vi "DatastructureTest.vi"() -> ()   [LabVIEW 2013, in "VI-Test.lvlib"]
uses:
  lib/VI-Test.lvlib
  classes/Datastructure/Report/Report.lvclass
  classes/Datastructure/Norm/Norm.lvclass
  classes/Datastructure/Test/Test.lvclass
  classes/Datastructure/Image/img.lvclass
  classes/Datastructure/Setup/Setup.lvclass
  classes/Datastructure/Device/Device.lvclass
  Main/controls/Data.ctl
  Main/controls/State.ctl
  classes/Devices/emTestCWS500N/EMTestCWS500N.lvclass
  classes/Devices/CEG4500/CEG4500.lvclass
  classes/Devices/Tektronix RSA5106A/Tektronix RSA5106A.lvclass
  classes/Devices/DeviceInterface/Devices.ctl
  classes/Tests/TestInterface/Tests.ctl
  lib/XML.lvlib
  lib/TreeRepresentation.lvlib
panel:
  in  "gelesen von XML":string(tree)
  in  "gelesen vom Baum":string(tree)
  out "Fehler (Ausgang)":errorcluster
  in  "gelesen von Datenstruktur":string(tree)
  out "Report (Ausgang)":refnum<class "Report.lvclass">
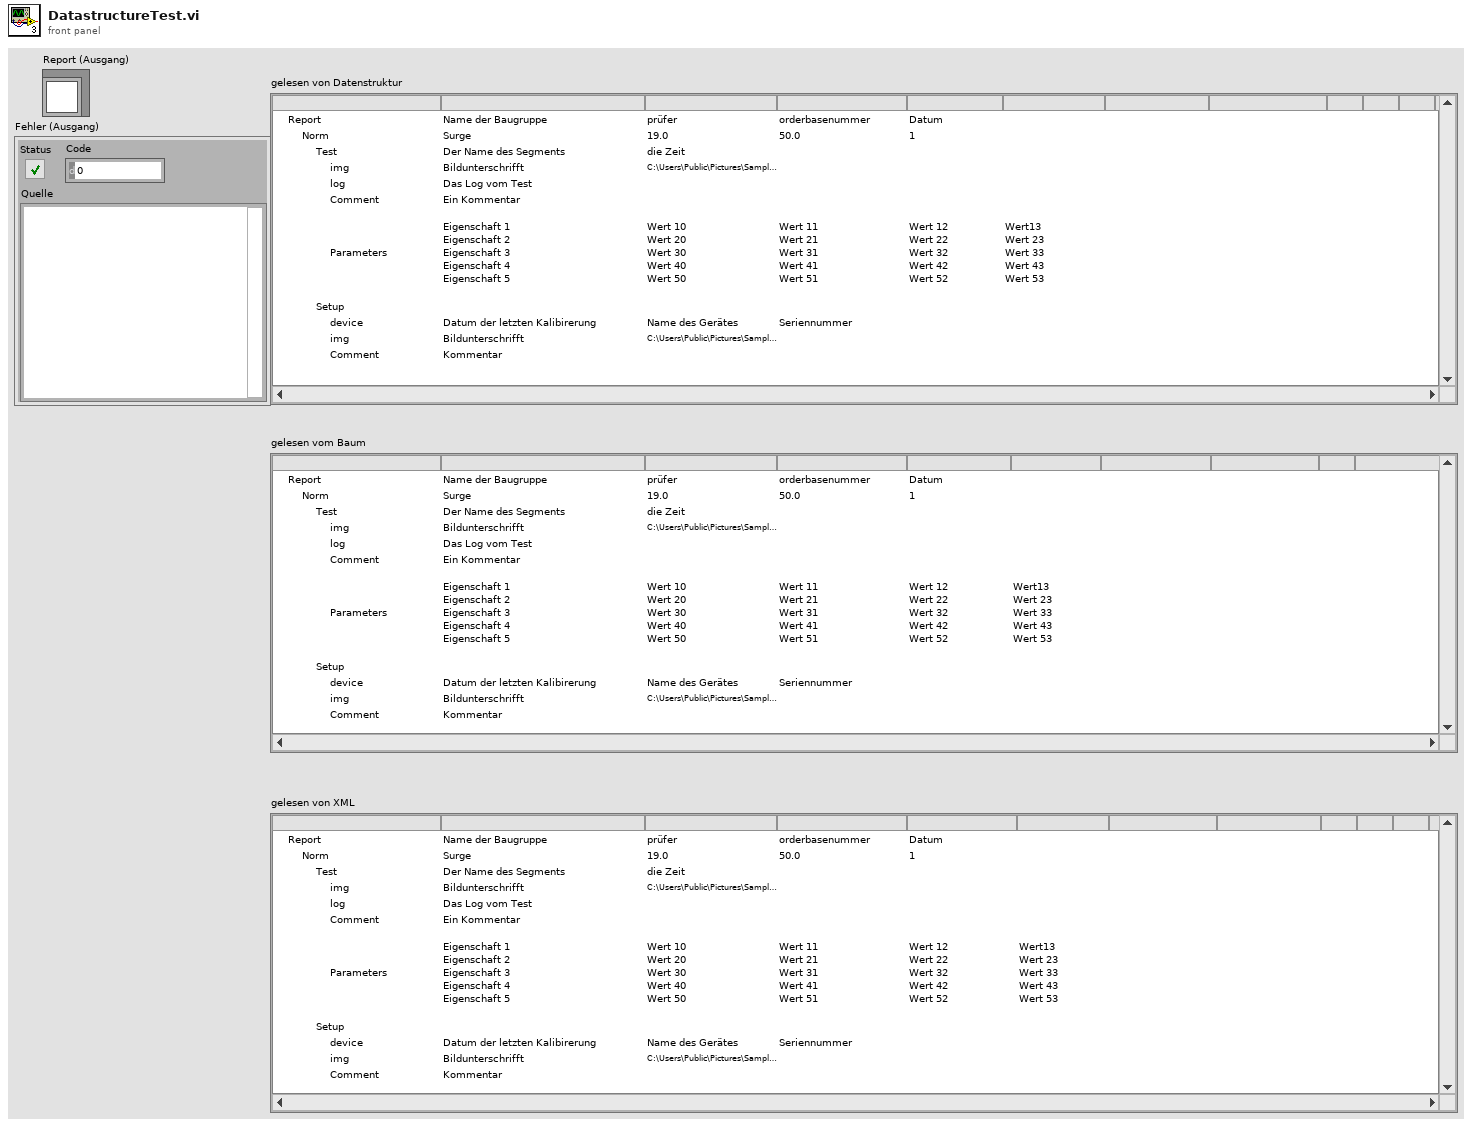
[diagram p1: front panel]
types:
  T1 = typedef "Data.ctl" = cluster{"Report.lvclass":refnum<class "Report.lvclass">, "Norm":string, "last State":T2, "Norm ID":i32, "parameter":string[][], "EMTestCWS500N.lvclass":refnum<class "EMTestCWS500N.lvclass">, "CEG4500.lvclass":refnum<class "CEG4500.lvclass">, "Tektronix RSA5106A.lvclass":refnum<class "Tektronix RSA5106A.lvclass">, "erfolgreich":bool, "log":string, "Kommentar":string, "Device Enum":T3, "Test Enum":T4, "debug":bool}
  T2 = typedef "State.ctl" = enum16{"create Pdf", "load Report", "save Report", "do Test", "CDN Kalibrierung", "enter Report Parameters", "new Test", "Protokoll", "read Tree", "update Tree", "Fehler", "Initialize", "Wait for Event", "Exit"}
  T3 = typedef "Devices.ctl" = enum16{"unbekannt", "Tektronix RSA5106A", "emTestCWS500N", "CEG-4500"}
  T4 = typedef "Tests.ctl" = enum16{"unbekannt", "Störaussendung", "Burst", "ESD", "Surge", "Spannungseinbruch", "HF-Felder"}
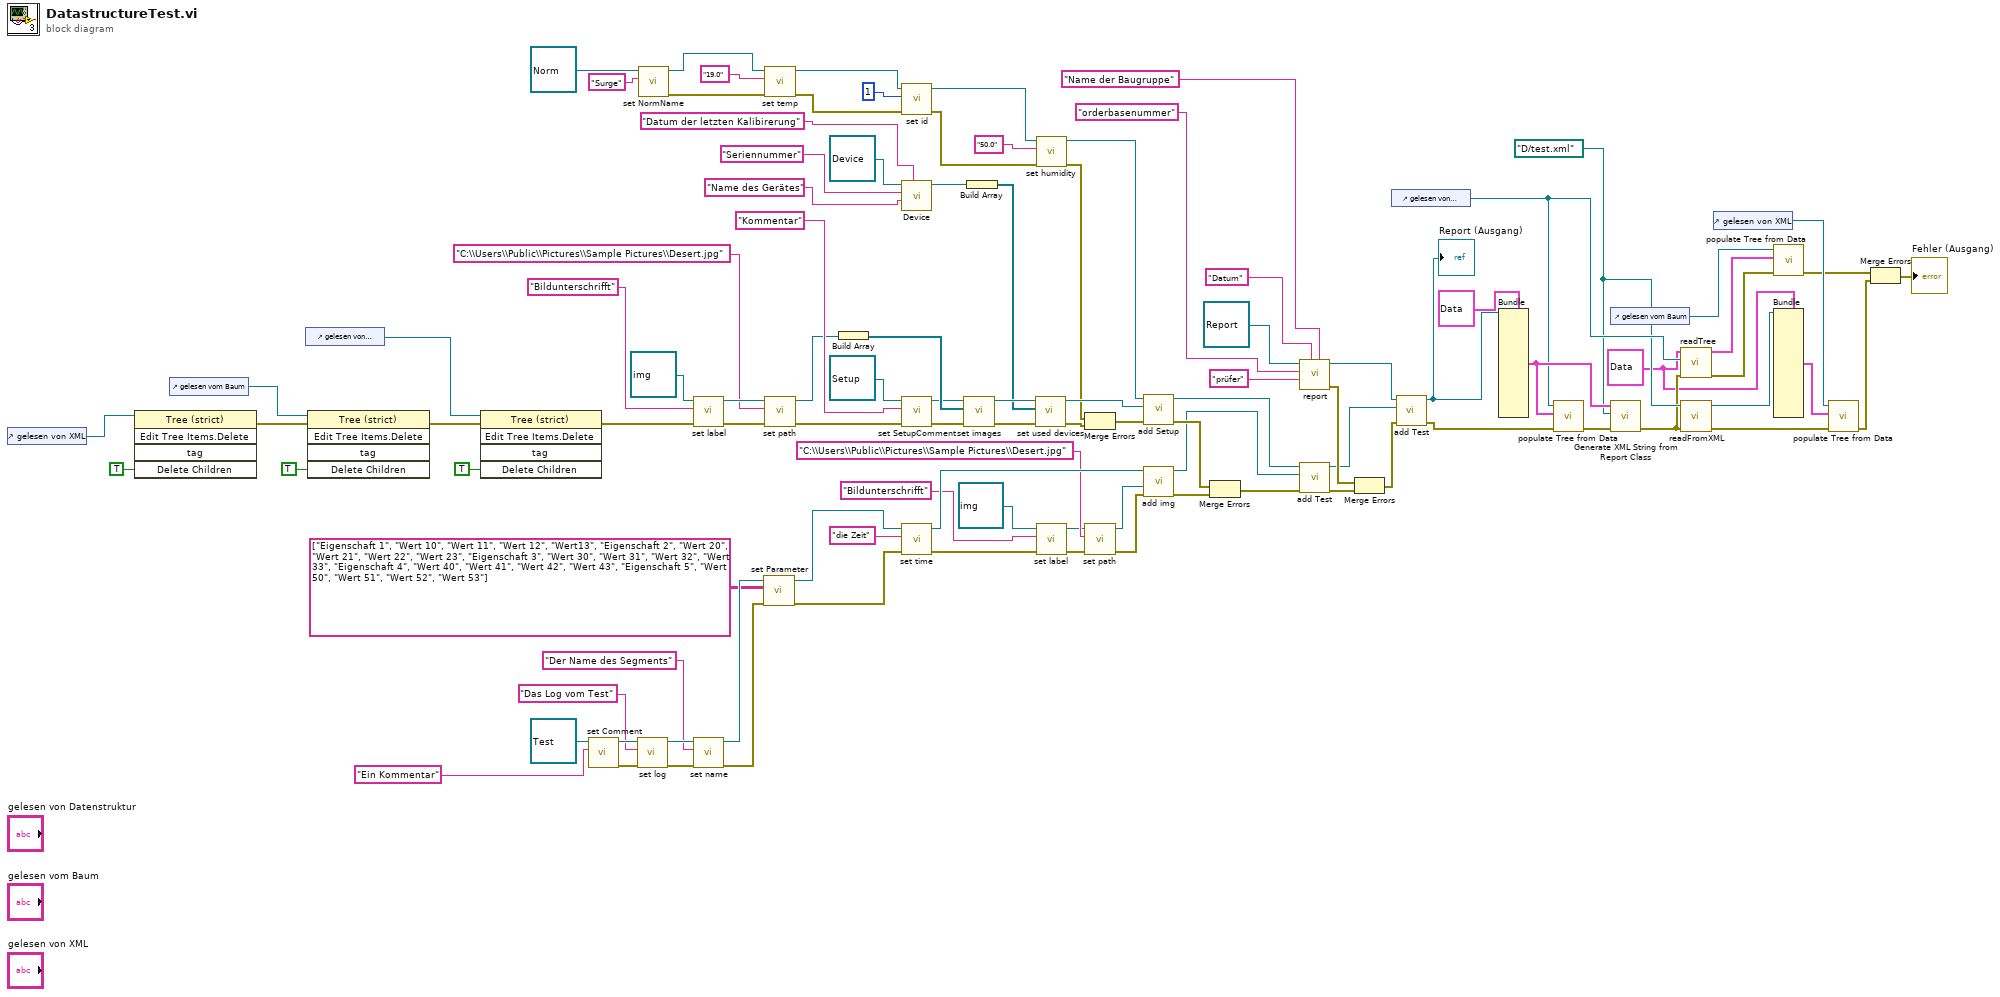
[diagram p0: block diagram]
diagram:
  w26 = T1 {"Report.lvclass"=refnum, "Norm"="", "last State"=enum."do Test", "Norm ID"=0, "parameter"=[], "EMTestCWS500N.lvclass"=refnum, "CEG4500.lvclass"=refnum, "Tektronix RSA5106A.lvclass"=refnum, "erfolgreich"=FALSE, "log"="", "Kommentar"="", "Device Enum"=enum."unbekannt", "Test Enum"=enum."unbekannt", "debug"=FALSE} ("Data out (Eingang)")
  w28 = path "D:/test.xml" ("Dateipfad (Dialog verwenden)")
  n1 = control-ref of="gelesen von XML"() -> (w14:refnum<vi>)
  n2 = invoke class="Tree (strict)" method="Edit Tree Items.Delete"(reference=w14, "Delete Children"=TRUE ("Unterobjekte löschen?")) -> (error out=w10:errorcluster)  [unwired: 3 in, 4 out]
  n3 = control-ref of="gelesen vom Baum"() -> (w13:refnum<vi>)
  n4 = control-ref of="gelesen von Datenstruktur"() -> (w18:refnum<vi>)
  n5 = invoke class="Tree (strict)" method="Edit Tree Items.Delete"(reference=w13, error in=w10, "Delete Children"=TRUE ("Unterobjekte löschen?")) -> (error out=w11:errorcluster)  [unwired: 2 in, 4 out]
  n6 = invoke class="Tree (strict)" method="Edit Tree Items.Delete"(reference=w18, error in=w11, "Delete Children"=TRUE ("Unterobjekte löschen?")) -> (error out=w12:errorcluster)  [unwired: 2 in, 4 out]
  n7 = call-dynamic "set Comment.vi"("Comment"="Ein Kommentar", "Test (Eingang)"=refnum<class "Test.lvclass"> refnum ("Segment.lvclass")) -> ("error out"=w80:errorcluster, "Test (Ausgang)"=w87:refnum<class "Test.lvclass">)  [unwired: 8 in]
  n8 = call-dynamic "set log.vi"("error in (no error)"=w80, "log"="Das Log vom Test", "Test (Eingang)"=w87) -> ("error out"=w81:errorcluster, "Test (Ausgang)"=w86:refnum<class "Test.lvclass">)  [unwired: 7 in]
  n9 = call-dynamic "set NormName.vi"("name"="Surge", "Norm (Eingang)"=refnum<class "Norm.lvclass"> refnum ("Test.lvclass")) -> ("error out"=w3:errorcluster, "Norm (Ausgang)"=w4:refnum<class "Norm.lvclass">)  [unwired: 8 in]
  n10 = call-dynamic "set label.vi"("error in (no error)"=w12, "label"="Bildunterschrifft", "img (Eingang)"=refnum<class "img.lvclass"> refnum ("img.lvclass")) -> ("error out"=w65:errorcluster, "img (Ausgang)"=w64:refnum<class "img.lvclass">)  [unwired: 7 in]
  n11 = call-dynamic "set name.vi"("error in (no error)"=w81, "name"="Der Name des Segments", "Test (Eingang)"=w86) -> ("error out"=w82:errorcluster, "Test (Ausgang)"=w85:refnum<class "Test.lvclass">)  [unwired: 7 in]
  n12 = call-dynamic "set Parameter.vi"("error in (no error)"=w82, "Parameter"=string[][] [["Eigenschaft 1", "Wert 10", "Wert 11", "Wert 12", "Wert13"], ["Eigenschaft 2", "Wert 20", "Wert 21", "Wert 22", "Wert 23"], ["Eigenschaft 3", "Wert 30", "Wert 31", "Wert 32", "Wert 33"], ["Eigenschaft 4", "Wert 40", "Wert 41", "Wert 42", "Wert 43"], ["Eigenschaft 5", "Wert 50", "Wert 51", "Wert 52", "Wert 53"]], "Test (Eingang)"=w85) -> ("error out"=w83:errorcluster, "Test (Ausgang)"=w84:refnum<class "Test.lvclass">)  [unwired: 7 in]
  n13 = call-dynamic "set temp.vi"("error in (no error)"=w3, "temp"="19.0", "Norm (Eingang)"=w4) -> ("error out"=w94:errorcluster, "Norm (Ausgang)"=w96:refnum<class "Norm.lvclass">)  [unwired: 7 in]
  n14 = call-dynamic "set path.vi"("error in (no error)"=w65, "path"="C:\\Users\\Public\\Pictures\\Sample Pictures\\Desert.jpg", "img (Eingang)"=w64) -> ("error out"=w40:errorcluster, "img (Ausgang)"=w57:refnum<class "img.lvclass">)  [unwired: 7 in]
  n15 = Build Array(w57) -> (w56:refnum<class "img.lvclass">[])
  n16 = call-dynamic "set id.vi"("error in (no error)"=w94, "id"=1, "Test (Eingang)"=w96) -> ("error out"=w93:errorcluster, "Test (Ausgang)"=w95:refnum<class "Norm.lvclass">)  [unwired: 7 in]
  n17 = call-dynamic "Device.vi"("last calibration"="Datum der letzten Kalibirerung", "Name"="Name des Gerätes", "serial"="Seriennummer", "Device Eingang"=refnum<class "Device.lvclass"> refnum ("Device.lvclass")) -> ("Device Ausgang"=w48:refnum<class "Device.lvclass">)  [unwired: 6 in, 1 out]
  n18 = call-dynamic "set SetupComment.vi"("error in (no error)"=w40, "Comment"="Kommentar", "Setup (Eingang)"=refnum<class "Setup.lvclass"> refnum ("Setup.lvclass")) -> ("error out"=w58:errorcluster, "Setup (Ausgang)"=w55:refnum<class "Setup.lvclass">)  [unwired: 7 in]
  n19 = call-dynamic "set time.vi"("error in (no error)"=w83, "time"="die Zeit", "Test (Eingang)"=w84) -> ("error out"=w66:errorcluster, "Test (Ausgang)"=w74:refnum<class "Test.lvclass">)  [unwired: 7 in]
  n20 = call-dynamic "set images.vi"("error in (no error)"=w58, "images"=w56, "Setup (Eingang)"=w55) -> ("error out"=w54:errorcluster, "Setup (Ausgang)"=w53:refnum<class "Setup.lvclass">)  [unwired: 7 in]
  n21 = Build Array(w48) -> (w47:refnum<class "Device.lvclass">[])
  n22 = call-dynamic "set used devices.vi"("error in (no error)"=w54, "used devices"=w47, "Setup (Eingang)"=w53) -> ("error out"=w44:errorcluster, "Setup (Ausgang)"=w46:refnum<class "Setup.lvclass">)  [unwired: 7 in]
  n23 = call-dynamic "set humidity.vi"("error in (no error)"=w93, "humidity"="50.0", "Test (Eingang)"=w95) -> ("error out"=w45:errorcluster, "Test (Ausgang)"=w89:refnum<class "Norm.lvclass">)  [unwired: 7 in]
  n24 = call-dynamic "set label.vi"("error in (no error)"=w66, "label"="Bildunterschrifft", "img (Eingang)"=refnum<class "img.lvclass"> refnum ("img.lvclass")) -> ("error out"=w67:errorcluster, "img (Ausgang)"=w70:refnum<class "img.lvclass">)  [unwired: 7 in]
  n25 = Merge Errors(w45, w44) -> (w43:errorcluster)
  n26 = call-dynamic "set path.vi"("error in (no error)"=w67, "path"="C:\\Users\\Public\\Pictures\\Sample Pictures\\Desert.jpg", "img (Eingang)"=w70) -> ("error out"=w68:errorcluster, "img (Ausgang)"=w69:refnum<class "img.lvclass">)  [unwired: 7 in]
  n27 = call-dynamic "add Setup.vi"("error in (no error)"=w43, "Setup"=w46, "Test Eingang"=w89) -> ("error out"=w42:errorcluster, "Test Ausgang"=w9:refnum<class "Norm.lvclass">)  [unwired: 7 in]
  n28 = call-dynamic "add img.vi"("error in (no error)"=w68, "img.lvclass"=w69, "Test (Eingang)"=w74) -> ("error out"=w41:errorcluster, "Test (Ausgang)"=w8:refnum<class "Test.lvclass">)  [unwired: 6 in]
  n29 = Merge Errors(w42, w41) -> (w7:errorcluster)
  n30 = call-dynamic "report.vi"("Rname"="Name der Baugruppe", "date"="Datum", "pruefer"="prüfer", "obnr"="orderbasenummer", "Report in"=refnum<class "Report.lvclass"> refnum ("Report.lvclass")) -> ("error out"=w39:errorcluster, "Report out"=w101:refnum<class "Report.lvclass">)  [unwired: 5 in]
  n31 = call-dynamic "add Test.vi"("error in (no error)"=w7, "Test.lvclass"=w8, "Test Eingang"=w9) -> ("error out"=w6:errorcluster, "Test Ausgang"=w5:refnum<class "Norm.lvclass">)  [unwired: 7 in]
  n32 = Merge Errors(w39, w6) -> (w38:errorcluster)
  n33 = control-ref of="gelesen von Datenstruktur"() -> (w32:refnum<vi>)
  n34 = call-dynamic "add Test.vi"("error in (no error)"=w38, "Norm.lvclass"=w5, "Report (Eingang)"=w101) -> ("error out"=w34:errorcluster, "Report (Ausgang)"=w36:refnum<class "Report.lvclass">)  [unwired: 7 in]
  "Report (Ausgang)" <- w36
  n35 = Bundle(cluster=T1 {"Report.lvclass"=refnum, "Norm"="", "last State"=enum."do Test", "Norm ID"=0, "parameter"=[], "EMTestCWS500N.lvclass"=refnum, "CEG4500.lvclass"=refnum, "Tektronix RSA5106A.lvclass"=refnum, "erfolgreich"=FALSE, "log"="", "Kommentar"="", "Device Enum"=enum."unbekannt", "Test Enum"=enum."unbekannt", "debug"=FALSE} ("Data"), "Report.lvclass"=w36) -> (w35:T1)  [unwired: 13 in]
  n36 = call "populate Tree from Data.vi"("error in (no error)"=w34, "Data"=w35, "reference"=w32) -> ("error out"=w33:errorcluster)  [unwired: 6 in]
  n37 = control-ref of="gelesen vom Baum"() -> (w30:refnum<vi>)
  n38 = call "Generate XML String from Report Class.vi"("error in (no error)"=w33, "Dateipfad (Dialog verwenden)"=w28, "Daten"=w35) -> ("Fehler (Ausgang)"=w27:errorcluster)  [unwired: 8 in]
  n39 = call "readTree.vi"("Fehler (Eingang, kein Fehler)"=w27, "Tree ref"=w32, "Data out (Eingang)"=w26) -> ("error out"=w29:errorcluster, "Data out (Ausgang)"=w31:T1)  [unwired: 7 in]
  n40 = call "readFromXML.vi"("error in (no error)"=w27, "file path (use dialog)"=w28) -> ("error out"=w22:errorcluster, "Report (Ausgang)"=w25:refnum<class "Report.lvclass">)  [unwired: 8 in]
  n41 = control-ref of="gelesen von XML"() -> (w23:refnum<vi>)
  n42 = call "populate Tree from Data.vi"("error in (no error)"=w29, "Data"=w31, "reference"=w30) -> ("error out"=w20:errorcluster)  [unwired: 6 in]
  n43 = Bundle(cluster=w26, "Report.lvclass"=w25) -> (w24:T1)  [unwired: 13 in]
  n44 = call "populate Tree from Data.vi"("error in (no error)"=w22, "Data"=w24, "reference"=w23) -> ("error out"=w21:errorcluster)  [unwired: 6 in]
  n45 = Merge Errors(w20, w21) -> (→"Fehler (Ausgang)":errorcluster)
